vi "Resource_Menu list.vi"() -> (1 "endofvalues":string="endofvalues", 2 "Resource_Menu list":string[][](array[string])=[["Control Label", "Control Caption", "Value 1", "Value 2", "Value 3", "Value 4", "Value 5"], ["Reference Source", "Reference", "Internal Ref", "External Ref/Aux", "External Ref/DIO", "External Ref/Trigger", ""]])   [LabVIEW 2016]
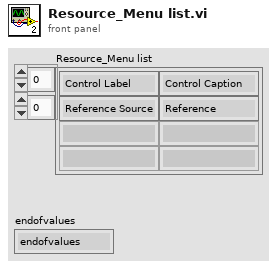
[diagram p1: front panel]
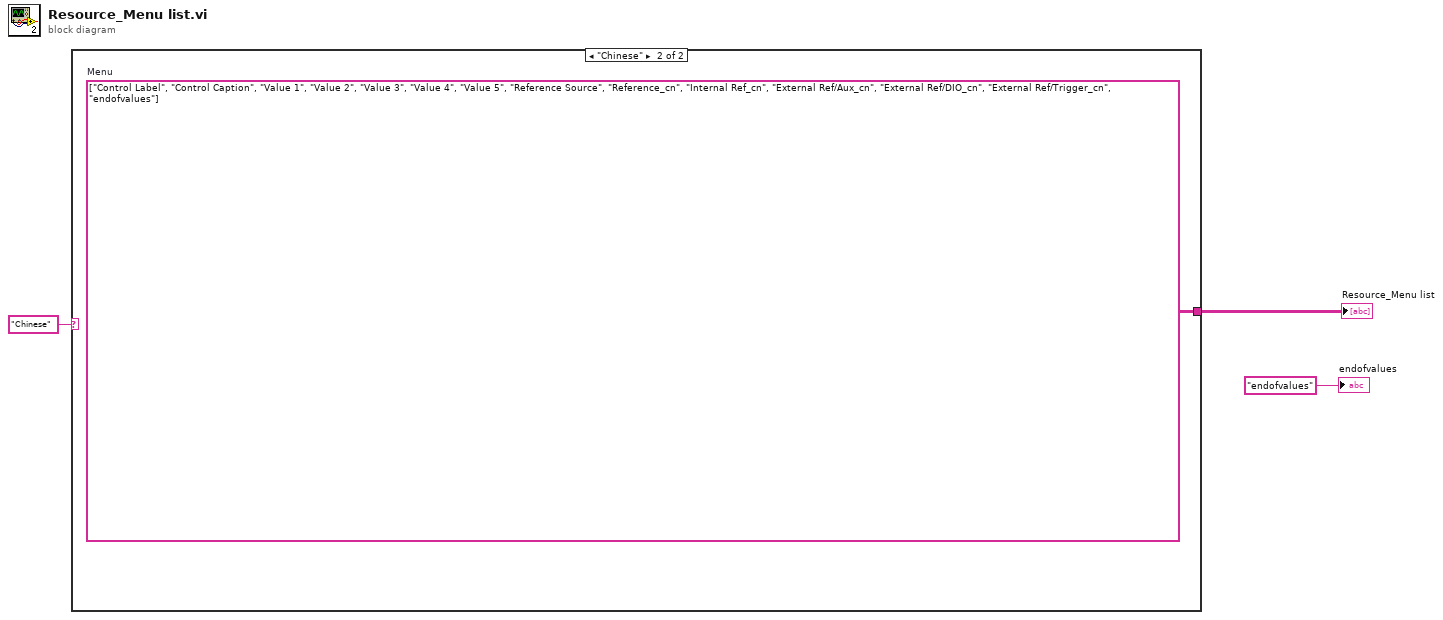
[diagram p0: block diagram]
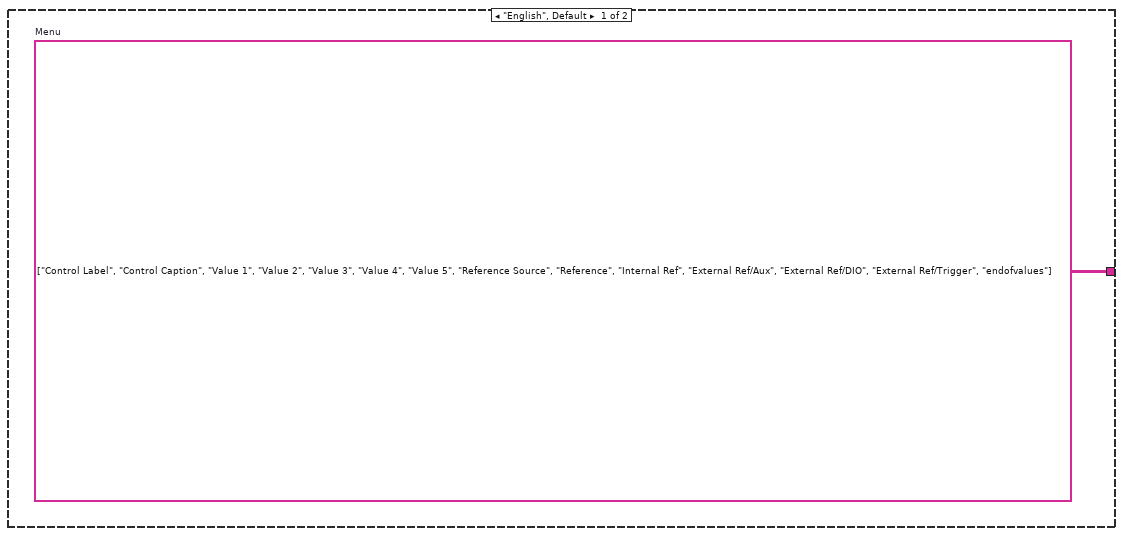
[diagram p2: hidden frame]
diagram:
  n1 = case shown="\"Chinese\"" "Chinese" {
    tunnel: [w4 w5] -> w3
    frame "English", Default {
      w4 = string[][] [["Control Label", "Control Caption", "Value 1", "Value 2", "Value 3", "Value 4", "Value 5"], ["Reference Source", "Reference", "Internal Ref", "External Ref/Aux", "External Ref/DIO", "External Ref/Trigger", "endofvalues"]]  # Menu
    }
    frame "Chinese" {
      w5 = string[][] [["Control Label", "Control Caption", "Value 1", "Value 2", "Value 3", "Value 4", "Value 5"], ["Reference Source", "Reference_cn", "Internal Ref_cn", "External Ref/Aux_cn", "External Ref/DIO_cn", "External Ref/Trigger_cn", "endofvalues"]]  # Menu
    }
  }
  "Resource_Menu list" <- w3
  "endofvalues" <- "endofvalues"
